vi "Identify.vi"(8 "error in (no error)":errorcluster, 11 "Config Parser SPI_3W in":refnum<class "Config Parser SPI_3W.lvclass">) -> (0 "error out":errorcluster, 2 "Plugin is Valid":bool, 3 "Config Parser SPI_3W out":refnum<class "Config Parser SPI_3W.lvclass">)   [LabVIEW 2018, in "Config Parser SPI_3W.lvlib" / "Config Parser SPI_3W.lvclass"]
uses:
  Config Parser SPI_3W.lvclass
  C:/P4 Workspace/PC Client/Solutions/5g_eap/trunk/1.0/HiSi5GmmWave/Pattern_Gen_Tool/Interfaces/File Parser Interface.lvlibp/Interfaces/File Parser Interface/File Parser Interface.lvclass
  Ctls/Protocol Type.ctl
  Interfaces/File Parser Interface.lvlibp/Interfaces/File Parser Interface/Read Protocol Type.vi
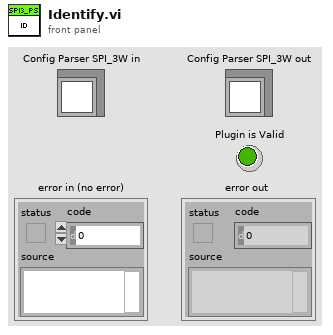
[diagram p1: front panel]
types:
  T1 = typedef "Protocol Type.ctl" = enum16{"BML_LS", "BML_HS", "SPI_3W", "SPI_4W"}
  T2 = typedef "File Parser Interface.lvlibp/Protocol Type.ctl" = enum16{"BML_LS", "BML_HS", "SPI_3W", "SPI_4W"}
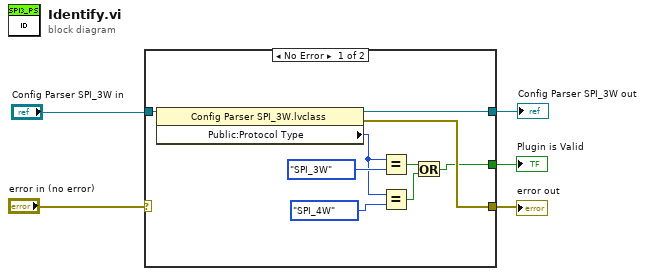
[diagram p0: block diagram]
diagram:
  n1 = case shown="No Error" "error in (no error)" {
    selector: "error in (no error)" -> [_ w15]
    tunnel: "Config Parser SPI_3W in" -> [w14 w16]
    tunnel: [w6 _] -> w1
    tunnel: [w12 w15] -> w3
    tunnel: [w11 w16] -> w2
    frame No Error {
      n2 = property class="Config Parser SPI_3W.lvclass"(reference=w14) -> (reference out=w11:refnum<class "Config Parser SPI_3W.lvclass">, error out=w12:errorcluster, "Public:Protocol Type"=w10:T2)  [unwired: 1 in]
      n3 = Equal?(x=w10, y=Protocol_Type."SPI_3W") -> (x = y?=w8:bool)
      n4 = Equal?(x=w10, y=Protocol_Type."SPI_4W") -> (x = y?=w7:bool)
      n5 = Or(x=w8, y=w7) -> (x .or. y?=w6:bool)
    }
    frame Error {
    }
  }
  "error out" <- w3
  "Config Parser SPI_3W out" <- w2
  "Plugin is Valid" <- w1
